vi "remove channel from configuration.vi"(8 "error in":errorcluster, 10 "TBM channel in":refnum<class "TBM channel.lvclass">, 11 "TDMS datalogger configuration in":refnum<class "TDMS datalogger configuration.lvclass">) -> (0 "error out":errorcluster, 3 "TDMS datalogger configuration out":refnum<class "TDMS datalogger configuration.lvclass">)   [LabVIEW 2013, in "TDMS datalogger configuration.lvclass"]
uses:
  TDMS datalogger configuration.lvclass
  <vilib>/NI/Tag Bus Module Framework/channel/TBM channel.lvclass
  <vilib>/NI/Tag Bus/tag/tag descriptor.lvclass/tag descriptor.ctl
  TDMS datalogger configuration.lvclass/TDMS datalogger configuration.ctl
  Read channels.vi
  Write channels.vi
  <vilib>/NI/Tag Bus/tag/read tag name.vi
  <vilib>/NI/Tag Bus/tag/tag descriptor.lvclass
  <vilib>/NI/Tag Bus Module Framework/root configuration/TBM configuration.lvclass
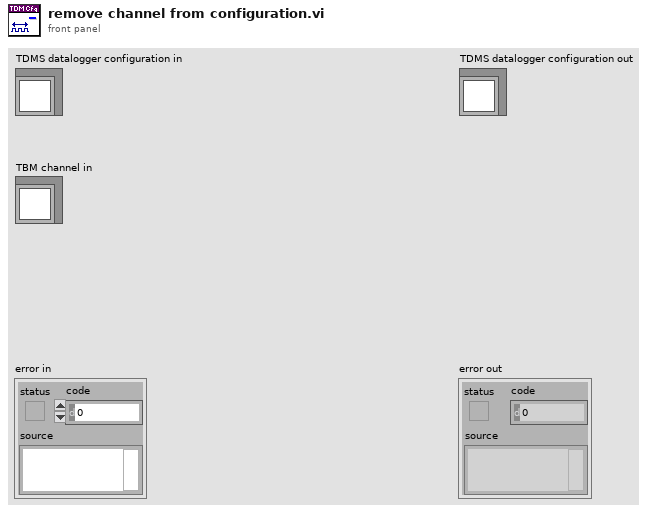
[diagram p1: front panel]
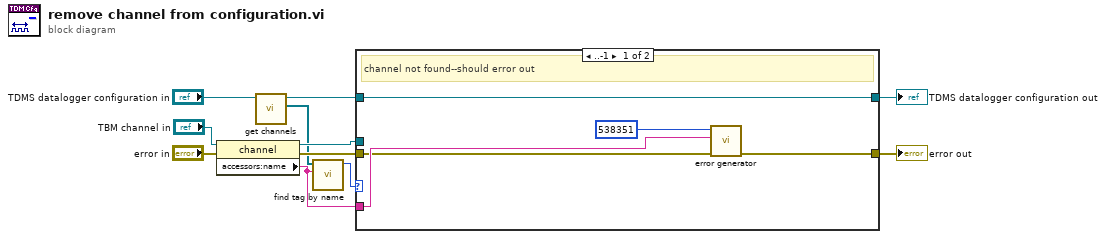
[diagram p0: block diagram]
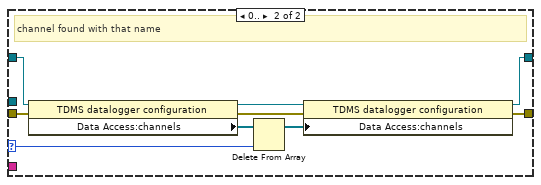
[diagram p2: hidden frame]
diagram:
  n1 = property class="channel"(reference="TBM channel in", error in="error in") -> (reference out=w10:refnum<class "TBM channel.lvclass">, error out=w9:errorcluster, "accessors:name"=w2:string)
  n2 = call-dynamic "get channels.vi"("module configuration in"="TDMS datalogger configuration in") -> ("channels"=w3:refnum<class "TBM channel.lvclass">[], "module configuration out"=w11:refnum<class "TDMS datalogger configuration.lvclass">)  [unwired: 9 in]
  n3 = call <vilib>:"find tag by name.vi"("name"=w2, "tags in"=w3) -> ("index"=w1:i32)  [unwired: 9 in]
  n4 = case shown="..-1" w1 {
    selector: w1 -> [_ w17]
    tunnel: [w16 w21] -> w4
    tunnel: w2 -> [w14 _]
    tunnel: w9 -> [w13 w25]
    tunnel: w11 -> [w12 w24]
    tunnel: w10 -> [_ _]
    tunnel: [w12 w20] -> w5
    frame ..-1 {
      # "channel not found--should error out"
      n5 = call <vilib>:"error generator.vi"("error in"=w13, "append error message"=w14, "error code (0)"=538351) -> ("error out"=w16:errorcluster)  [unwired: 8 in]
    }
    frame 0.. {
      # "channel found with that name"
      n6 = property class="TDMS datalogger configuration"(reference=w24, error in=w25) -> (reference out=w23:refnum<class "TDMS datalogger configuration.lvclass">, error out=w22:errorcluster, "Data Access:channels"=w19:refnum<class "TBM channel.lvclass">[])
      n7 = Delete From Array(array=w19, index=w17) -> (array with subset deleted=w18:refnum<class "TBM channel.lvclass">[])  [unwired: 1 in, 1 out]
      n8 = property class="TDMS datalogger configuration"(reference=w23, error in=w22, "Data Access:channels"=w18) -> (reference out=w20:refnum<class "TDMS datalogger configuration.lvclass">, error out=w21:errorcluster)
    }
  }
  "error out" <- w4
  "TDMS datalogger configuration out" <- w5
